vi "WriteRead Data.vi"(7 "SPI Device":refnum<class "SPI Device.lvclass">, 8 "error in (no error)":errorcluster, 10 "Write Data":string, 11 "Session In":refnum<class "Session.lvclass">) -> (0 "error out":errorcluster, 1 "Read Data":string, 3 "Session Out":refnum<class "Session.lvclass">)   [LabVIEW 2020, in "CTI.lvlib" / "SPI Device.lvclass"]
uses:
  SPI Device.lvclass
  SPI Device.lvclass/SPI Device.ctl
  SPI/SPI.lvclass
  Session/Session.lvclass
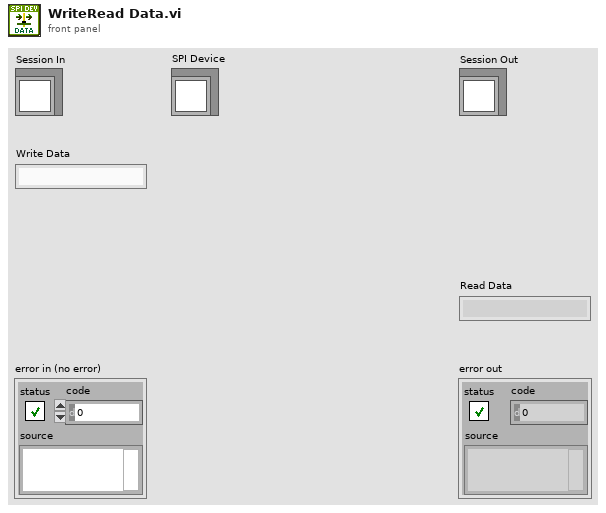
[diagram p1: front panel]
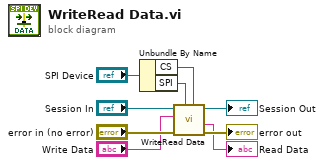
[diagram p0: block diagram]
diagram:
  n1 = Unbundle By Name("SPI Device") -> ("CS"=w3:refnum<class "SPI CS.lvclass">, "SPI"=w4:refnum<class "SPI.lvclass">)
  n2 = call "WriteRead Data.vi"("CS (None)"=w3, "SPI"=w4, "error in (no error)"="error in (no error)", "Write Data"="Write Data", "Session In"="Session In") -> ("error out"=→"error out":errorcluster, "Read Data"=→"Read Data":string, "Session Out"=→"Session Out":refnum<class "Session.lvclass">)  [unwired: 4 in]
